vi "population_manipulations.vi"(0 "RF Power":dbl, 1 "Microwave on":bool, 2 "Zero Ensemble Out":dbl[](array[numeric]), 3 "Zero Level on":bool, 4 "rho- array in":dbl[](array[numeric]), 5 "Thermally Connect Zero Ensemble":bool, 6 "Zero Ensemble Power":dbl, 8 "RF Indicator":bool, 9 "rho+ array in":dbl[](array[numeric]), 10 "Drive Zero Level Down":bool, 11 "rho0 array in":dbl[](array[numeric]), 12 "AFP Efficiency":dbl, 13 "rho- array in":dbl[](array[numeric]), 14 "Numeric":i32, 15 "rho+ array in":dbl[](array[numeric]), 16 "RF Proportional to Intensity":bool, 17 "rho0 array in":dbl[](array[numeric]), 18 "Numeric 2":i32, 19 "rho0 decay in":dbl[](array[numeric])) -> (20 "Zero ensemble out":dbl[](array[numeric]), 21 "rho0 out":dbl[](array[numeric]), 22 "rho+ out":dbl[](array[numeric]), 23 "rho- out":dbl[](array[numeric]))   [LabVIEW 2018]
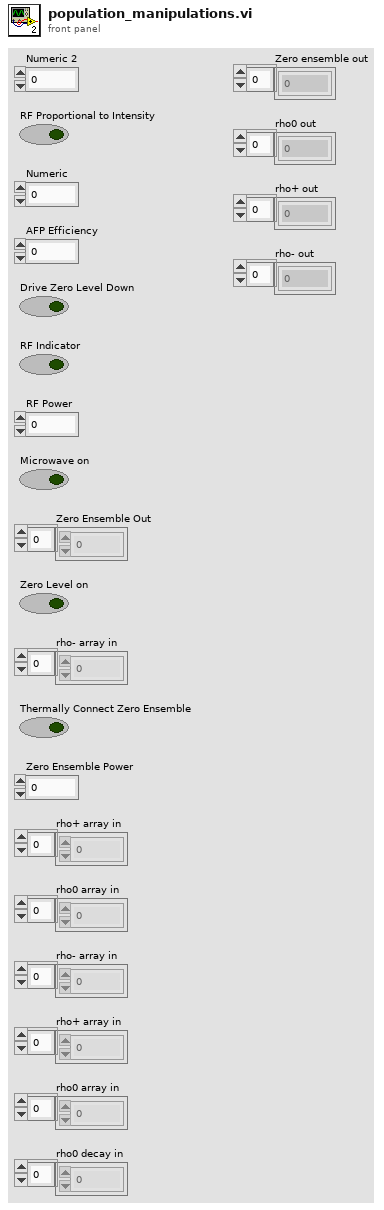
[diagram p1: front panel]
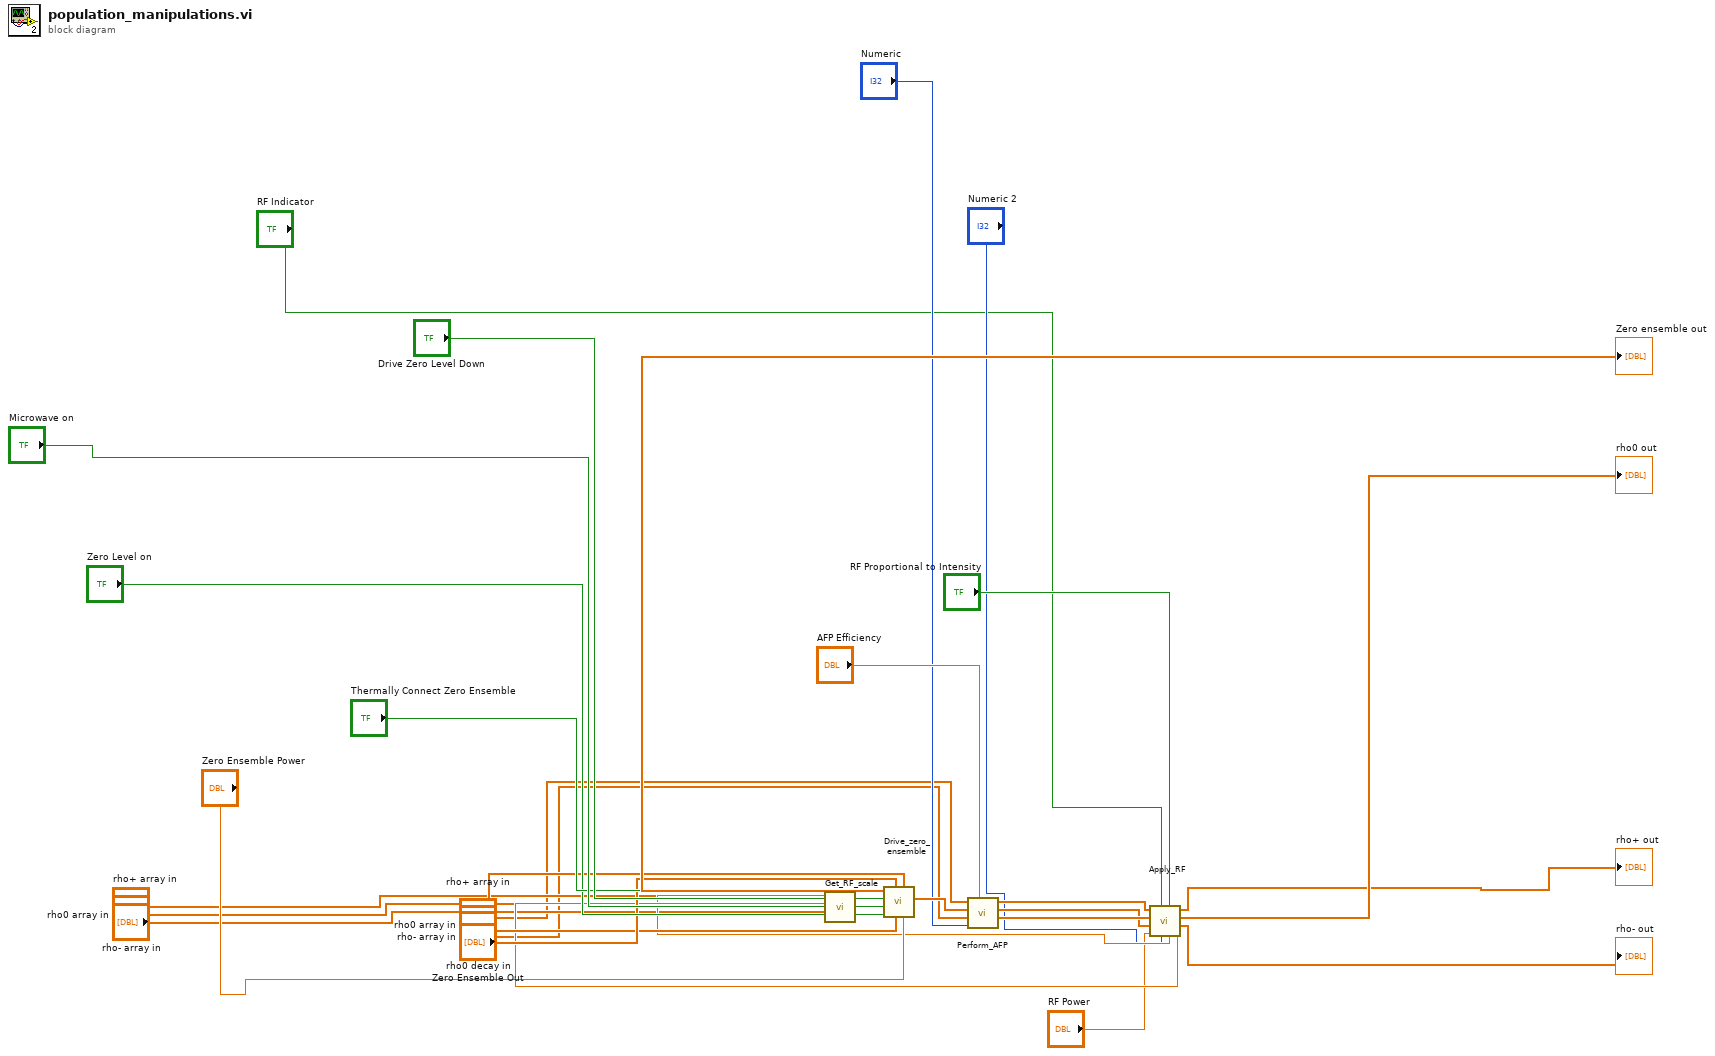
[diagram p0: block diagram]
diagram:
  n1 = call "Get_RF_scale.vi"("rho-"="rho- array in", "rho0"="rho0 array in", "rho+"="rho+ array in") -> ("I-  index out"=w11:dbl, "I+ index out"=w10:dbl)  [unwired: 7 in]
  n2 = call "Drive_zero_ensemble.vi"("Zero ensemble power in"="Zero Ensemble Power", "rho0 in"="rho0 array in", "rho0 decay in"="rho0 decay in", "Zero ensemble in"="Zero Ensemble Out", "Drive Zero Ensemble Up"="Zero Level on", "Microwave on"="Microwave on", "Drive Zero Ensemble Down"="Drive Zero Level Down", "Thermal connection"="Thermally Connect Zero Ensemble") -> ("rho0 out"=w23:dbl[], "Zero ensemble out"=→"Zero ensemble out":dbl[])  [unwired: 2 in]
  n3 = call "Perform_AFP.vi"("AFP Efficiency"="AFP Efficiency", "AFP Target"="Numeric", "rho-"="rho- array in", "rho0"=w23, "rho+"="rho+ array in") -> ("rho- out"=w19:dbl[], "rho0 out"=w18:dbl[], "rho+ out"=w17:dbl[])  [unwired: 4 in]
  n4 = call "Apply_RF.vi"("I- index"=w11, "I+ index"=w10, "RF Proportional to intensity"="RF Proportional to Intensity", "RF Target Position"="Numeric 2", "RF indicator"="RF Indicator", "RF Power"="RF Power", "rho0"=w18, "rho-"=w19, "rho+"=w17) -> ("rho- out"=→"rho- out":dbl[], "rho0 out"=→"rho0 out":dbl[], "rho+ out"=→"rho+ out":dbl[])
